vi "SImple PID.vi"(5 "Desired Setpoint":dbl, 6 "I Windup Limit":dbl, 7 "Current Setpoint":dbl, 9 "D":dbl, 10 "I":dbl, 11 "P":dbl) -> (2 "output":dbl)   [LabVIEW 2017]
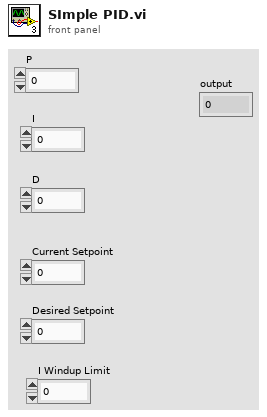
[diagram p1: front panel]
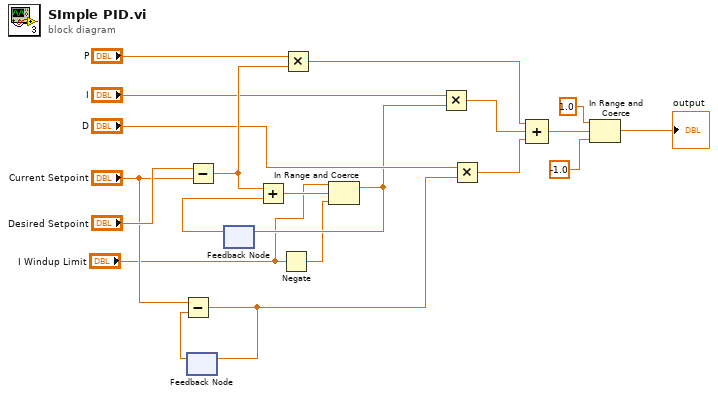
[diagram p0: block diagram]
diagram:
  n1 = feedback #1() -> (w12:dbl)  [unwired: 1 in]
  n2 = Subtract(x="Current Setpoint", y=w12) -> (x-y=w11:dbl)
  n3 = feedback-in #1(w11) -> ()
  n4 = Subtract(x="Desired Setpoint", y="Current Setpoint") -> (x-y=w18:dbl)
  n5 = feedback #2() -> (w17:dbl)  [unwired: 1 in]
  n6 = Add(x=w18, y=w17) -> (x+y=w4:dbl)
  n7 = Negate(x="I Windup Limit") -> (-x=w2:dbl)
  n8 = Multiply(x="P", y=w18) -> (x*y=w19:dbl)
  n9 = In Range and Coerce(upper limit="I Windup Limit", x=w4, lower limit=w2) -> (coerced(x)=w3:dbl)  [unwired: 1 out]
  n10 = feedback-in #2(w3) -> ()
  n11 = Multiply(x="I", y=w3) -> (x*y=w15:dbl)
  n12 = Multiply(x="D", y=w11) -> (x*y=w13:dbl)
  n13 = Compound Arithmetic op=ADD(w19, w15, w13) -> (w8:dbl)
  n14 = In Range and Coerce(upper limit=1.0, x=w8, lower limit=-1.0) -> (coerced(x)=→"output":dbl)  [unwired: 1 out]
